vi "Obj to TreeItem.vi"(8 "error in (no error)":errorcluster, 11 "BetterTreeItem in":refnum<class "BetterItem.lvclass">) -> (0 "error out":errorcluster, 2 "Tree Control Item":T1, 3 "BetterTreeItem out":refnum<class "BetterItem.lvclass">)   [LabVIEW 2020, in "BetterDragAndDrop.lvlib" / "BetterItem.lvclass"]
uses:
  BetterItem.lvclass
  SubVIs/TreeItem.ctl
  BetterItem.lvclass/BetterItem.ctl
  BetterTreeHandle/BetterTreeHandle.lvclass
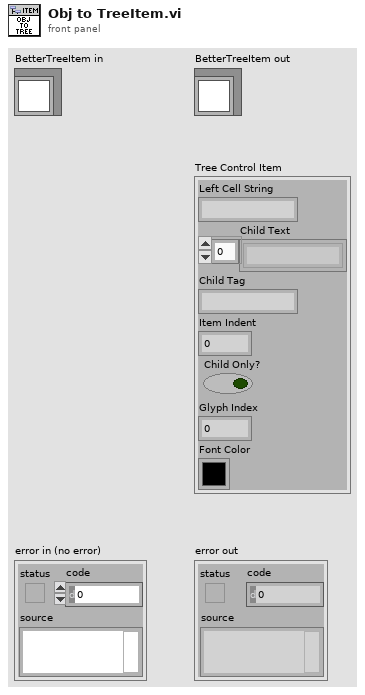
[diagram p1: front panel]
types:
  T1 = typedef "BetterDragAndDrop.lvlib/BetterTreeHandle.lvclass/TreeItem.ctl" = cluster{"Left Cell String":string, "Child Text":string[], "Child Tag":string, "Item Indent":i32, "Child Only?":bool, "Glyph Index":i32, "Font Color":u32}
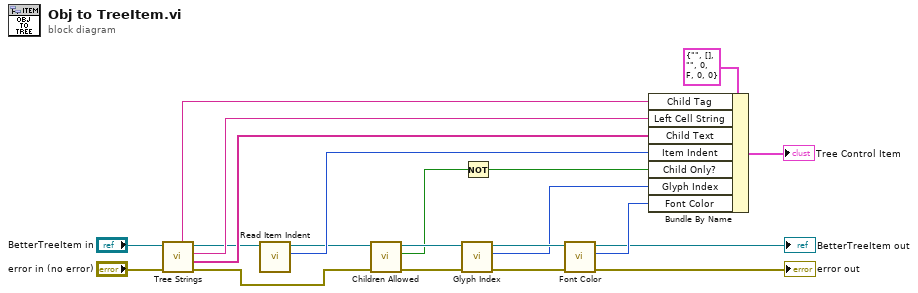
[diagram p0: block diagram]
diagram:
  n1 = call-dynamic "Tree Strings.vi"("error in (no error)"="error in (no error)", "BetterItem in"="BetterTreeItem in") -> ("error out"=w6:errorcluster, "Child Text"=w10:string[], "Left Cell String"=w11:string, "BetterItem out"=w9:refnum<class "BetterItem.lvclass">, "Child Tag"=w12:string)  [unwired: 5 in]
  n2 = call "Read Item Indent.vi"("BetterTreeItem in"=w9) -> ("Item Indent"=w19:i32, "BetterTreeItem out"=w15:refnum<class "BetterItem.lvclass">)  [unwired: 9 in]
  n3 = call-dynamic "Children Allowed.vi"("error in (no error)"=w6, "BetterTreeItem in"=w15) -> ("error out"=w5:errorcluster, "Child allowed?"=w2:bool, "BetterTreeItem out"=w14:refnum<class "BetterItem.lvclass">)  [unwired: 7 in]
  n4 = call-dynamic "Glyph Index.vi"("error in (no error)"=w5, "BetterItem in"=w14) -> ("error out"=w4:errorcluster, "Glyph Index"=w16:i32, "BetterItem out"=w17:refnum<class "BetterItem.lvclass">)  [unwired: 7 in]
  n5 = Not(x=w2) -> (.not. x?=w1:bool)
  n6 = call-dynamic "Font Color.vi"("error in (no error)"=w4, "BetterItem in"=w17) -> ("error out"=→"error out":errorcluster, "Font Color"=w18:u32, "BetterItem out"=→"BetterTreeItem out":refnum<class "BetterItem.lvclass">)  [unwired: 7 in]
  n7 = Bundle By Name(cluster=T1 {"Left Cell String"="", "Child Text"=[], "Child Tag"="", "Item Indent"=0, "Child Only?"=FALSE, "Glyph Index"=0, "Font Color"=0} ("Tree Control Item"), "Child Tag"=w12, "Left Cell String"=w11, "Child Text"=w10, "Item Indent"=w19, "Child Only?"=w1, "Glyph Index"=w16, "Font Color"=w18) -> (→"Tree Control Item":T1)
